vi "Start Processes.vi"(8 "error in (no error)":errorcluster, 9 "Timeout [ms] (-1)":i32=-1, 11 "Rig in":refnum<class "Application.lvclass">) -> (0 "error out":errorcluster, 3 "Rig out":refnum<class "Application.lvclass">)   [LabVIEW 2020, in "Application.lvclass"]
uses:
  Application.lvclass
  Application.lvclass/Application.ctl
  Process/Process.lvclass
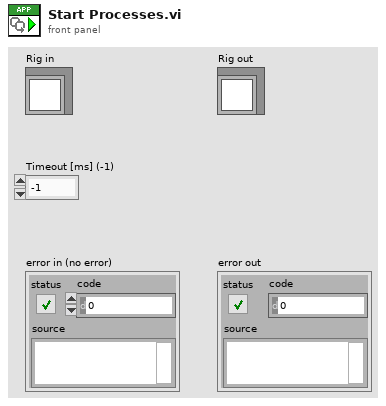
[diagram p1: front panel]
types:
  T1 = typedef "Process.lvclass/Lifecycle State.ctl" = enum16{"Uninitialized", "Initialized", "Started", "Running", "Stopped", "Finished"}
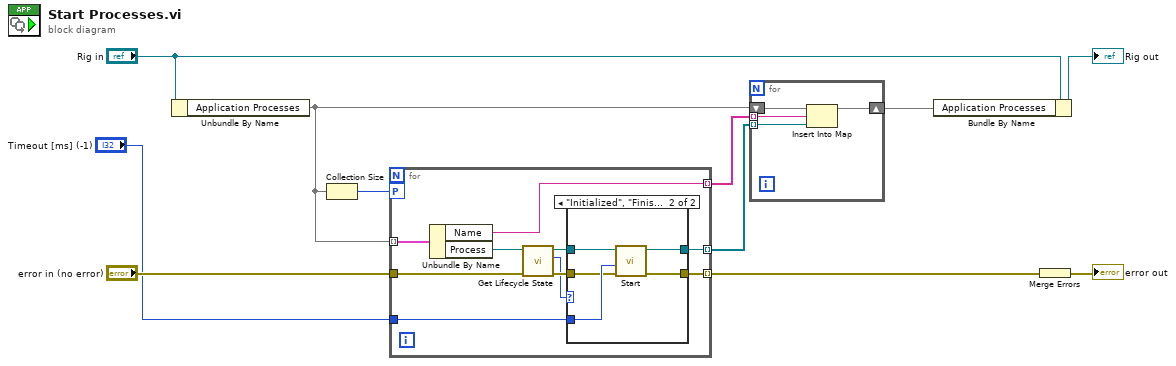
[diagram p0: block diagram]
diagram:
  n1 = Unbundle By Name("Rig in") -> ("Application Processes"=w4:map{string, refnum<class "Process.lvclass">})
  n2 = Collection Size(1:w4) -> (0:w6:i32)
  n3 = for {
    tunnel: w4 -> [w19] mode=indexing
    tunnel: "error in (no error)" -> [w20]
    tunnel: [w21] -> w10 mode=indexing
    workers-P: w6 -> [_]
    tunnel: "Timeout [ms] (-1)" -> [w18]
    tunnel: [w17] -> w2 mode=indexing
    tunnel: [w16] -> w1 mode=indexing
    n4 = Unbundle By Name(w19) -> ("Name"=w17:string, "Process"=w14:refnum<class "Process.lvclass">)
    n5 = call "Get Lifecycle State.vi"("error in (no error)"=w20, "Process In"=w14) -> ("error out"=w15:errorcluster, "Lifecycle State"=w12:T1, "Process Out"=w13:refnum<class "Process.lvclass">)  [unwired: 6 in, 1 out]
    n6 = case shown="\"Initialized\", \"Finished\"" w12 {
      tunnel: [w22 w28] -> w21
      tunnel: w18 -> [_ w27]
      tunnel: [w23 w26] -> w16
      tunnel: w15 -> [w22 w25]
      tunnel: w13 -> [w23 w24]
      frame "Uninitialized", Default {
      }
      frame "Initialized", "Finished" {
        n7 = call "Start.vi"("error in (no error)"=w25, "Timeout [ms] (-1)"=w27, "Process In"=w24) -> ("error out"=w28:errorcluster, "Process Out"=w26:refnum<class "Process.lvclass">)  [unwired: 7 in]
      }
    }
  }
  n8 = for {
    shift-right: [w31] -> w3
    shift-left: w4 -> [w32]
    tunnel: w2 -> [w30] mode=indexing
    tunnel: w1 -> [w29] mode=indexing
    n9 = Insert Into Map(map in=w32, key=w30, value=w29) -> (map out=w31:map{string, refnum<class "Process.lvclass">})  [unwired: 2 out]
  }
  n10 = Bundle By Name(cluster="Rig in", "Application Processes"=w3) -> (→"Rig out":refnum<class "Application.lvclass">)
  n11 = Merge Errors(w10) -> (→"error out":errorcluster)
